vi "DDFL_Controller_v31mai.vi"(0 "K":dbl[](array[numeric]), 1 "q_ref":dbl[](array[numeric]), 2 "q1":dbl, 3 "q2":dbl, 4 "q3":dbl, 5 "q4":dbl, 7 "K1":dbl, 9 "K2":dbl, 11 "K3":dbl, 13 "K4":dbl) -> (16 "u_out":dbl)   [LabVIEW 2021]
uses:
  <vilib>/Analysis/baseanly.llb/Real A x B.vi
  <vilib>/Analysis/Matrix/Numeric/Conversions/Matrix To Array - RM.vi
  <vilib>/Analysis/Matrix/Numeric/Conversions/Array To Matrix - RA2.vi
  <vilib>/Analysis/Matrix/NI_Matrix.lvlib
  <vilib>/Analysis/NI_AALBase.lvlib
panel:
  out "Control input u":dbl(graph)
  out "Gamma(q)":dbl(graph)
  out "Etta(q)":dbl(graph)
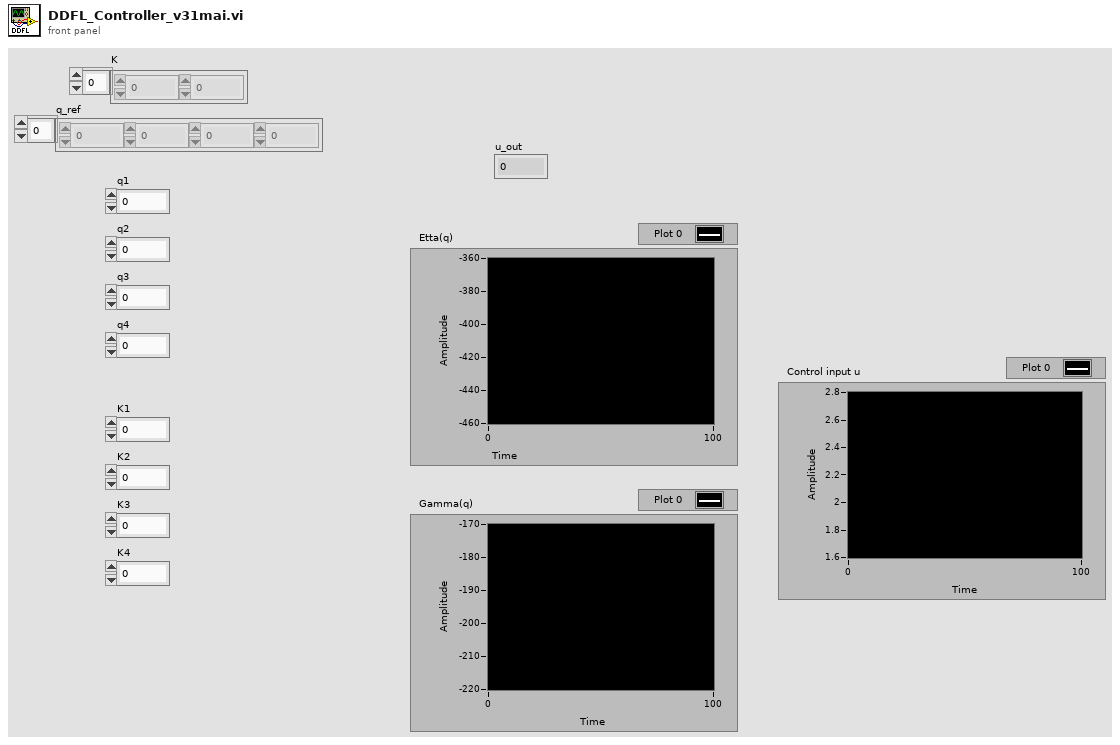
[diagram p1: front panel]
types:
  T1 = typedef "NI_Matrix.lvlib/RealMatrix.ctl" = dbl[][]
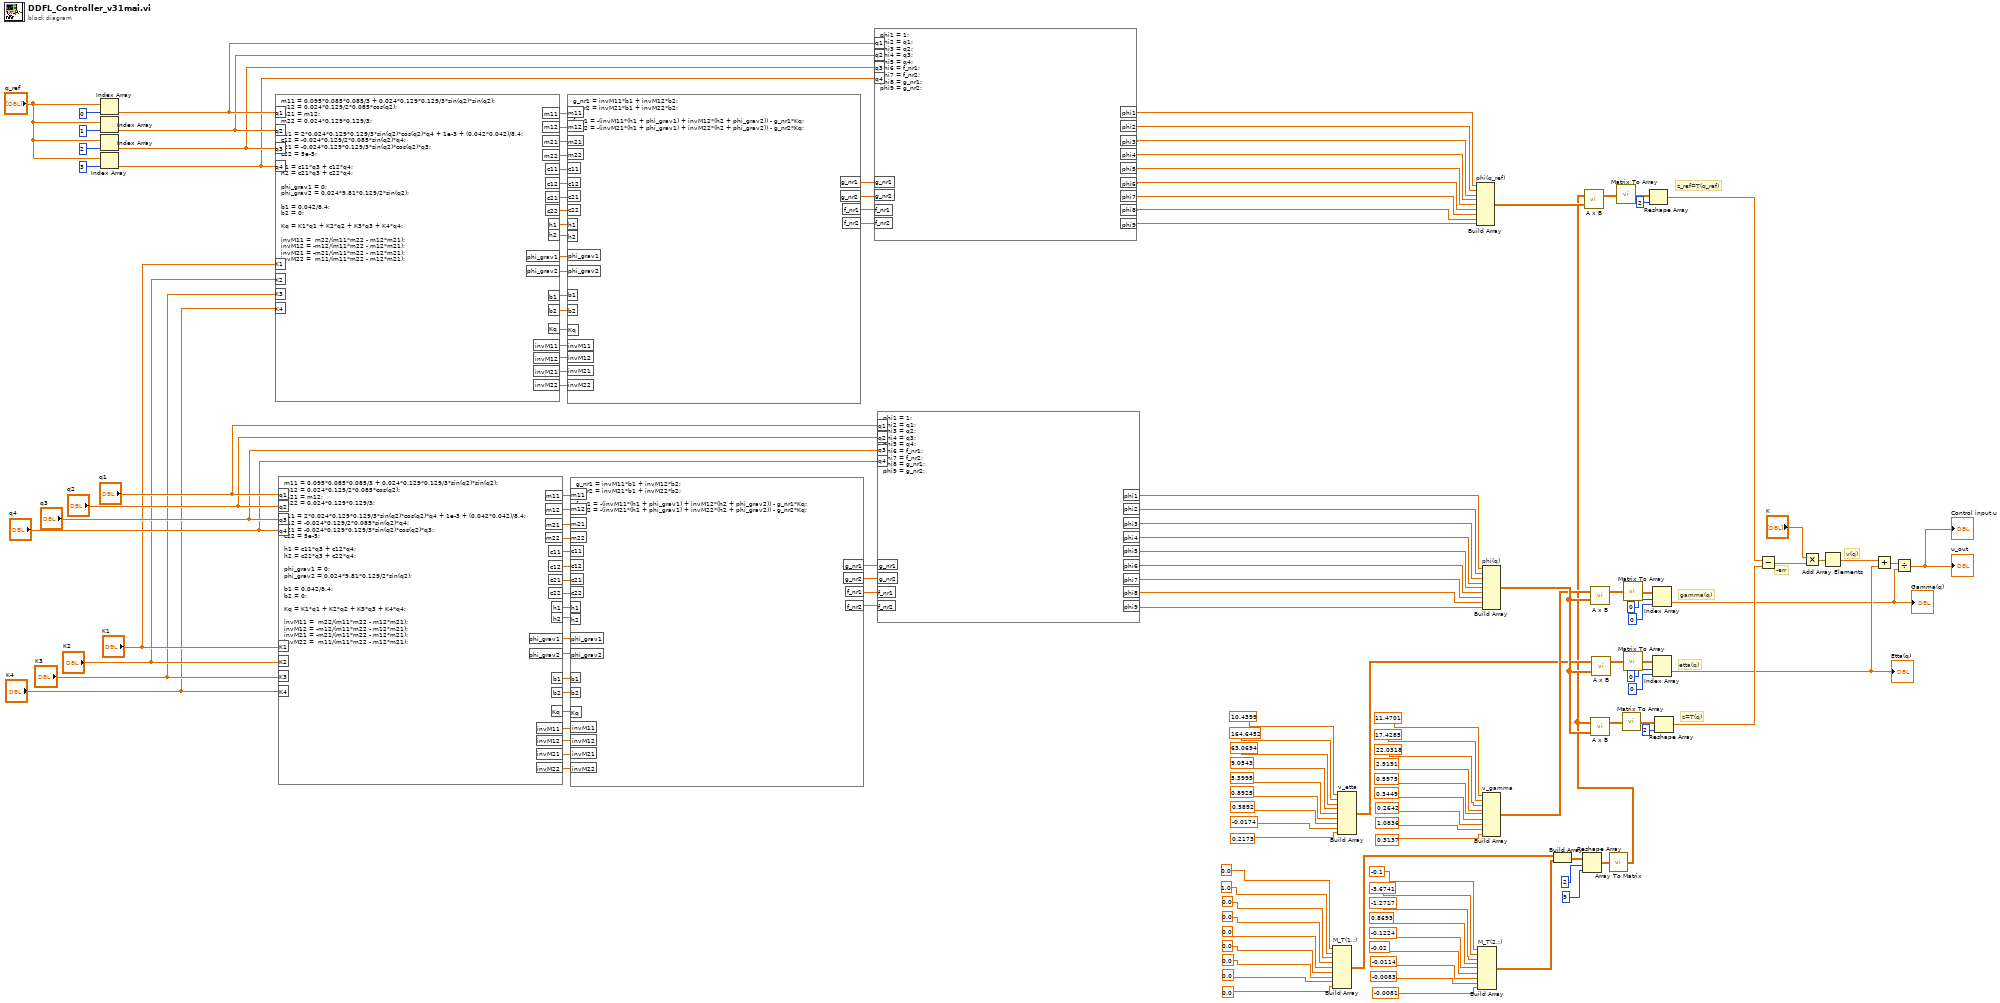
[diagram p0: block diagram]
diagram:
  # "z_ref=T(q_ref)"
  # "v(q)"
  # "-err"
  # "z=T(q)"
  # "etta(q)"
  # "gamma(q)"
  n1 = Index Array(array="q_ref", index=0 ("index 3")) -> (element=w15:dbl)
  n2 = Index Array(array="q_ref", index=1 ("index 4")) -> (element=w13:dbl)
  n3 = Index Array(array="q_ref", index=2 ("index 3")) -> (element=w12:dbl)
  n4 = Index Array(array="q_ref", index=3 ("index 4")) -> (element=w11:dbl)
  n5 = formula code="m11 = 0.095*0.085*0.085/3 + 0.024*0.129*0.129/3*sin(q2)*sin(q2);\nm12 = 0.024*0.129/2*0.085*cos(q2);\nm21 = m12;\nm22 = 0.024*0.129*0.129/3;\n\nc11 = 2*0.024*0.129*0.129/3*sin(q2)*cos(q2)*q4 + 1e-3 + (0.042*0.042)/8.4;\nc12 = -0.024*0.129/2*0.085*sin(q2)*q4;\nc21 = -0.024*0.129*0.129/3*sin(q2)*cos(q2)*q3;\nc22 = 5e-5;\n\nh1 = c11*q3 + c12*q4;\nh2 = c21*q3 + c22*q4;\n\nphi_grav1 = 0;\nphi_grav2 = 0.024*9.81*0.129/2*sin(q2);\n\nb1 = 0.042/8.4;\nb2 = 0;\n\nKq = K1*q1 + K2*q2 + K3*q3 + K4*q4;\n\ninvM11 =  m22/(m11*m22 - m12*m21);\ninvM12 = -m12/(m11*m22 - m12*m21);\ninvM21 = -m21/(m11*m22 - m12*m21);\ninvM22 =  m11/(m11*m22 - m12*m21);"("q1"=w15, "q2"=w13, "q3"=w12, "q4"=w11, "K1"="K1", "K2"="K2", "K3"="K3", "K4"="K4") -> ("m11"=w57:dbl, "m12"=w56:dbl, "m21"=w55:dbl, "m22"=w54:dbl, "c11"=w53:dbl, "c12"=w52:dbl, "c21"=w51:dbl, "c22"=w50:dbl, "h1"=w49:dbl, "h2"=w48:dbl, "phi_grav1"=w47:dbl, "phi_grav2"=w46:dbl, "b1"=w45:dbl, "b2"=w44:dbl, "Kq"=w43:dbl, "invM11"=w42:dbl, "invM12"=w41:dbl, "invM21"=w40:dbl, "invM22"=w39:dbl)
  n6 = formula code="m11 = 0.095*0.085*0.085/3 + 0.024*0.129*0.129/3*sin(q2)*sin(q2);\nm12 = 0.024*0.129/2*0.085*cos(q2);\nm21 = m12;\nm22 = 0.024*0.129*0.129/3;\n\nc11 = 2*0.024*0.129*0.129/3*sin(q2)*cos(q2)*q4 + 1e-3 + (0.042*0.042)/8.4;\nc12 = -0.024*0.129/2*0.085*sin(q2)*q4;\nc21 = -0.024*0.129*0.129/3*sin(q2)*cos(q2)*q3;\nc22 = 5e-5;\n\nh1 = c11*q3 + c12*q4;\nh2 = c21*q3 + c22*q4;\n\nphi_grav1 = 0;\nphi_grav2 = 0.024*9.81*0.129/2*sin(q2);\n\nb1 = 0.042/8.4;\nb2 = 0;\n\nKq = K1*q1 + K2*q2 + K3*q3 + K4*q4;\n\ninvM11 =  m22/(m11*m22 - m12*m21);\ninvM12 = -m12/(m11*m22 - m12*m21);\ninvM21 = -m21/(m11*m22 - m12*m21);\ninvM22 =  m11/(m11*m22 - m12*m21);"("q1"="q1", "q2"="q2", "q3"="q3", "q4"="q4", "K1"="K1", "K2"="K2", "K3"="K3", "K4"="K4") -> ("m11"=w84:dbl, "m12"=w83:dbl, "m21"=w82:dbl, "m22"=w81:dbl, "c11"=w80:dbl, "c12"=w79:dbl, "c21"=w78:dbl, "c22"=w77:dbl, "h1"=w76:dbl, "h2"=w75:dbl, "phi_grav1"=w74:dbl, "phi_grav2"=w73:dbl, "b1"=w72:dbl, "b2"=w71:dbl, "Kq"=w70:dbl, "invM11"=w69:dbl, "invM12"=w68:dbl, "invM21"=w67:dbl, "invM22"=w66:dbl)
  n7 = formula code="g_nr1 = invM11*b1 + invM12*b2;\ng_nr2 = invM21*b1 + invM22*b2;\n\nf_nr1 = -(invM11*(h1 + phi_grav1) + invM12*(h2 + phi_grav2)) - g_nr1*Kq;\nf_nr2 = -(invM21*(h1 + phi_grav1) + invM22*(h2 + phi_grav2)) - g_nr2*Kq;"("m11"=w57, "m12"=w56, "m21"=w55, "m22"=w54, "invM11"=w42, "invM12"=w41, "invM21"=w40, "invM22"=w39, "c11"=w53, "c12"=w52, "c21"=w51, "c22"=w50, "h1"=w49, "h2"=w48, "phi_grav1"=w47, "phi_grav2"=w46, "b1"=w45, "b2"=w44, "Kq"=w43) -> ("g_nr1"=w38:dbl, "g_nr2"=w37:dbl, "f_nr1"=w36:dbl, "f_nr2"=w35:dbl)
  n8 = formula code="g_nr1 = invM11*b1 + invM12*b2;\ng_nr2 = invM21*b1 + invM22*b2;\n\nf_nr1 = -(invM11*(h1 + phi_grav1) + invM12*(h2 + phi_grav2)) - g_nr1*Kq;\nf_nr2 = -(invM21*(h1 + phi_grav1) + invM22*(h2 + phi_grav2)) - g_nr2*Kq;"("m11"=w84, "m12"=w83, "m21"=w82, "m22"=w81, "invM11"=w69, "invM12"=w68, "invM21"=w67, "invM22"=w66, "c11"=w80, "c12"=w79, "c21"=w78, "c22"=w77, "h1"=w76, "h2"=w75, "phi_grav1"=w74, "phi_grav2"=w73, "b1"=w72, "b2"=w71, "Kq"=w70) -> ("g_nr1"=w65:dbl, "g_nr2"=w64:dbl, "f_nr1"=w63:dbl, "f_nr2"=w62:dbl)
  n9 = formula code="phi1 = 1;\nphi2 = q1;\nphi3 = q2;\nphi4 = q3;\nphi5 = q4;\nphi6 = f_nr1;\nphi7 = f_nr2;\nphi8 = g_nr1;\nphi9 = g_nr2;"("q1"=w15, "q2"=w13, "q3"=w12, "q4"=w11, "g_nr1"=w38, "g_nr2"=w37, "f_nr1"=w36, "f_nr2"=w35) -> ("phi1"=w34:dbl, "phi2"=w33:dbl, "phi3"=w32:dbl, "phi4"=w31:dbl, "phi5"=w30:dbl, "phi6"=w29:dbl, "phi7"=w28:dbl, "phi8"=w27:dbl, "phi9"=w26:dbl)
  n10 = formula code="phi1 = 1;\nphi2 = q1;\nphi3 = q2;\nphi4 = q3;\nphi5 = q4;\nphi6 = f_nr1;\nphi7 = f_nr2;\nphi8 = g_nr1;\nphi9 = g_nr2;"("q1"="q1", "q2"="q2", "q3"="q3", "q4"="q4", "g_nr1"=w65, "g_nr2"=w64, "f_nr1"=w63, "f_nr2"=w62) -> ("phi1"=w93:dbl, "phi2"=w92:dbl, "phi3"=w91:dbl, "phi4"=w90:dbl, "phi5"=w89:dbl, "phi6"=w88:dbl, "phi7"=w87:dbl, "phi8"=w86:dbl, "phi9"=w85:dbl)
  n11 = Build Array "M_T(1,:)"(0.0, 1.0, 0.0, 0.0, 0.0, 0.0, 0.0, 0.0, 0.0) -> (w99:T1)
  n12 = Build Array "v_etta"(10.4399, 164.6452, 63.0694, 9.0543, 5.3995, 0.8925, 0.5892, -0.0174, 0.2173) -> (w142:T1)
  n13 = Build Array "phi(q_ref)"(w34, w33, w32, w31, w30, w29, w28, w27, w26) -> (w22:T1)
  n14 = Build Array "M_T(2,:)"(-0.1, -3.6741, -1.2717, 0.8693, -0.1224, -0.02, -0.0114, -0.0083, -0.0081) -> (w98:T1)
  n15 = Build Array "phi(q)"(w93, w92, w91, w90, w89, w88, w87, w86, w85) -> (w144:T1)
  n16 = Build Array "v_gamma"(11.4701, 17.4285, 22.0318, 2.9191, 0.5975, 0.3449, 0.2642, 1.0836, 0.3137) -> (w143:T1)
  n17 = Build Array(w99, w98) -> (w97:dbl[][][])
  n18 = Reshape Array(w97, 2, 9) -> (w94:dbl[][])
  n19 = call-poly <vilib>:"A x B.vi"("B"=w144, "A"=w143) -> ("A x B"=w138:T1)  [unwired: 1 out]
  n20 = call-poly <vilib>:"A x B.vi"("B"=w144, "A"=w142) -> ("A x B"=w133:T1)  [unwired: 1 out]
  n21 = call-poly <vilib>:"Array To Matrix.vi"("Real 2D Array"=w94) -> ("Real Matrix"=w21:T1)
  n22 = call-poly <vilib>:"A x B.vi"("B"=w22, "A"=w21) -> ("A x B"=w25:T1)  [unwired: 1 out]
  n23 = call-poly <vilib>:"A x B.vi"("B"=w144, "A"=w21) -> ("A x B"=w134:T1)  [unwired: 1 out]
  n24 = call-poly <vilib>:"Matrix To Array.vi"("Real Matrix"=w25) -> ("Real 2D Array"=w24:dbl[][])
  n25 = call-poly <vilib>:"Matrix To Array.vi"("Real Matrix"=w134) -> ("Real 2D Array"=w132:dbl[][])
  n26 = call-poly <vilib>:"Matrix To Array.vi"("Real Matrix"=w138) -> ("Real 2D Array"=w141:dbl[][])
  n27 = call-poly <vilib>:"Matrix To Array.vi"("Real Matrix"=w133) -> ("Real 2D Array"=w137:dbl[][])
  n28 = Reshape Array(w24, 2 ("dimension size")) -> (w20:dbl[])
  n29 = Index Array ("Index Array 2")(array=w141, index (row)=0 ("index 3"), index (col)=0 ("index 4")) -> (element=w2:dbl)
  "Gamma(q)" <- w2
  n30 = Index Array ("Index Array 2")(array=w137, index (row)=0 ("index 3"), index (col)=0 ("index 4")) -> (element=w3:dbl)
  "Etta(q)" <- w3
  n31 = Reshape Array(w132, 2 ("dimension size")) -> (w130:dbl[])
  n32 = Subtract(x=w20, y=w130) -> (x-y=w128:dbl[])
  n33 = Multiply(x="K", y=w128) -> (x*y=w126:dbl[])
  n34 = Add Array Elements(numeric array=w126) -> (sum=w125:dbl)
  n35 = Add(x=w125, y=w3) -> (x+y=w127:dbl)
  n36 = Divide(x=w127, y=w2) -> (x/y=→"u_out" →"Control input u":dbl)
